vi "If Error.vi"(9 "Result code (error if non-zero)":u32=999, 10 "error in (no error)":errorcluster, 11 "PQ Connection in":refnum<class "PQ Connection.lvclass">) -> (2 "error out":errorcluster, 3 "PQ Connection out":refnum<class "PQ Connection.lvclass">)   [LabVIEW 2015, in "PQ Connection.lvclass"]
uses:
  PQ Connection.lvclass
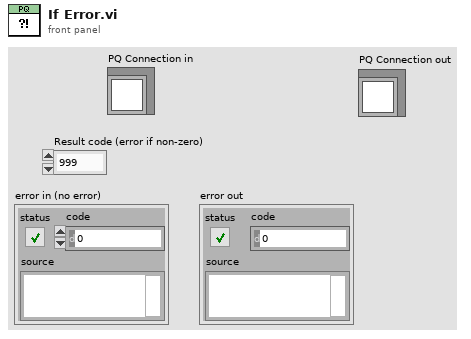
[diagram p1: front panel]
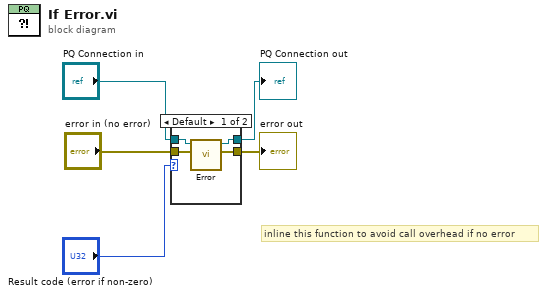
[diagram p0: block diagram]
diagram:
  # "inline this function to avoid call overhead if no error"
  n1 = case shown="Default" "Result code (error if non-zero)" {
    tunnel: "PQ Connection in" -> [w9 w11]
    tunnel: [w8 w11] -> w4
    tunnel: "error in (no error)" -> [w7 w10]
    tunnel: [w6 w10] -> w2
    frame Default {
      n2 = call "Error.vi"("error in (no error)"=w7, "PQ Connection in"=w9) -> ("error out"=w6:errorcluster, "PQ Connection out"=w8:refnum<class "PQ Connection.lvclass">)  [unwired: 8 in]
    }
    frame 0 {
    }
  }
  "error out" <- w2
  "PQ Connection out" <- w4
